vi "create default channels.vi"() -> (0 "error out":errorcluster, 1 "names":string[](array[string]), 2 "channels":refnum<class "TBM channel.lvclass">[](array[class]), 3 "module":refnum<class "UI Reference configuration old.lvclass">, 5 "instance identifier":string)   [LabVIEW 2014, in "UI reference module tests.lvlib"]
uses:
  UI reference module tests.lvlib
  <vilib>/NI/Tag Bus Module Framework/channel/channel classification.ctl
  <vilib>/NI/Tag Bus Module Framework/channel/TBM channel.lvclass
  module/configuration/UI Reference configuration old.lvclass
  <vilib>/NI/Configuration Framework/serializable configuration/NISE_CEF_serializable configuration.lvclass
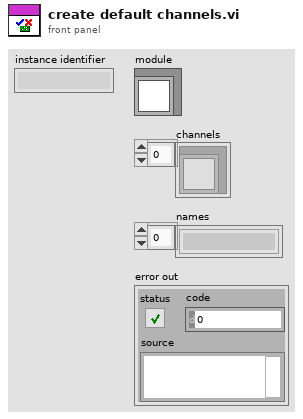
[diagram p1: front panel]
types:
  T1 = typedef "TBM channel.lvclass/channel classification.ctl" = enum16{"input data", "output data", "processing parameter", "processing result"}
  T2 = typedef "tag bus.lvlib/tag descriptor.lvclass/Data Type.ctl" = enum16{"Double", "Single", "I64", "I32", "I16", "I8", "U64", "U32", "U16", "U8", "Boolean", "String", "Array of Double", "Array of Single", "Array of I64", "Array of I32", "Array of I16", "Array of I8", "Array of U64", "Array of U32", "Array of U16", "Array of U8", "Array of Boolean", "Array of String"}
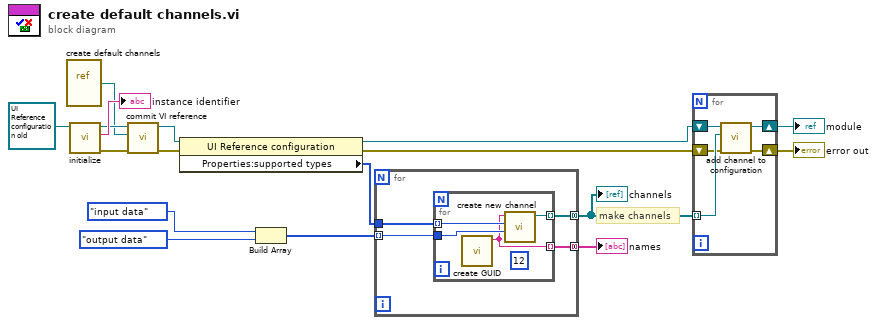
[diagram p0: block diagram]
diagram:
  # "make channels"
  n1 = vi-ref "create default channels.vi"() -> (w1:refnum<vi>)
  n2 = call <vilib>:"initialize.vi"("configuration in"=refnum<class "UI Reference configuration old.lvclass"> refnum ("tag bus configurable plugin module configuration")) -> ("error out"=w15:errorcluster, "identifier"=→"instance identifier":string, "configuration out"=w3:refnum<class "UI Reference configuration old.lvclass">)  [unwired: 8 in]
  n3 = call "commit VI reference.vi"("error in"=w15, "VI Refnum in"=w1, "UI Reference configuration in"=w3) -> ("error out"=w4:errorcluster, "UI Reference configuration out"=w2:refnum<class "UI Reference configuration old.lvclass">)  [unwired: 6 in, 1 out]
  n4 = property class="UI Reference configuration"(reference=w2, error in=w4) -> (reference out=w8:refnum<class "UI Reference configuration old.lvclass">, error out=w14:errorcluster, "Properties:supported types"=w9:T2[])
  n5 = Build Array(channel_classification."input data" ("channel classification"), channel_classification."output data" ("channel classification")) -> (w7:T1[])
  n6 = for {
    tunnel: w7 -> [w21] mode=indexing
    tunnel: [w19] -> w12 mode=concatenating
    tunnel: w9 -> [w20]
    tunnel: [w18] -> w13 mode=concatenating
    n7 = for {
      tunnel: w21 -> [w24]
      tunnel: [w25] -> w19 mode=indexing
      tunnel: w20 -> [w23] mode=indexing
      tunnel: [w22] -> w18 mode=indexing
      (unwired) 12
      n8 = call <vilib>:"create GUID.vi"() -> ("uuid"=w22:string)  [unwired: 10 in, 1 out]
      n9 = call <vilib>:"create new channel.vi"("channel classification"=w24, "data type"=w23, "channel name"=w22) -> ("channel"=w25:refnum<class "TBM channel.lvclass">)  [unwired: 8 in]
    }
  }
  "names" <- w13
  "channels" <- w12
  n10 = for {
    tunnel: w12 -> [w28] mode=indexing
    shift-right: [w29] -> w11
    shift-left: w8 -> [w30]
    shift-right: [w26] -> w17
    shift-left: w14 -> [w27]
    n11 = call "add channel to configuration.vi"("error in"=w27, "channel"=w28, "UI Reference configuration in"=w30) -> ("error out"=w26:errorcluster, "UI Reference configuration out"=w29:refnum<class "UI Reference configuration old.lvclass">)  [unwired: 7 in]
  }
  "error out" <- w17
  "module" <- w11
